vi "high_field_probe_chopper.vi"() -> ()   [LabVIEW 2011]
uses:
  <vilib>/express/express arith-compare/Formula/XNode/ExpressFormulaBlockNode.xnode
  <vilib>/Analysis/NI_AAL_SigProc.lvlib
panel:
  out "Signal":dbl[](graph)
  in  "Set Probe Background":bool
  out "Probe Background":dbl[](graph)
  in  "peak threshold":dbl=0.01 format="%0.2f"
  out "Amplitudes":dbl[](array[numeric])
  in  "Fits?":bool
  out "Waveform Chart 2":dbl(graph)
  out "best fit parameters":dbl[](array[numeric])
  in  "Set Zero Peaks":bool
  out "Peak 2 Amp":dbl
  out "Peak 1 Amp":dbl
  out "Polarization":dbl
  out "Peak Ratio":dbl
  out "XY Graph":cluster{dbl[], dbl[]}[](graph)
  in  "Peak 2 at Zero":dbl=1.0
  in  "Peak 1 at Zero":dbl=1.0
  in  "fit parameters":dbl[](array[numeric])=[0.02, 0.3, 0.12, 0.005, 0.13, 0.012, 0.03, 1.4, 0.12]
  in  "stop":bool
  in  "Center Freq":dbl=1000.0
  in  "Voltage Sweep Range":i32=2
  out "Current Set Voltage":dbl
  in  "threshold":dbl=0.0005
  in  "rate":dbl=20000.0
  in  "number of samples":i32=500
  out "data":dynamicdata(graph)
  out "Waveform Chart":dbl(graph)
  out "amplitude":dbl
  out "frequency":dbl
  # "Height"
  # "Position"
  # "Width"
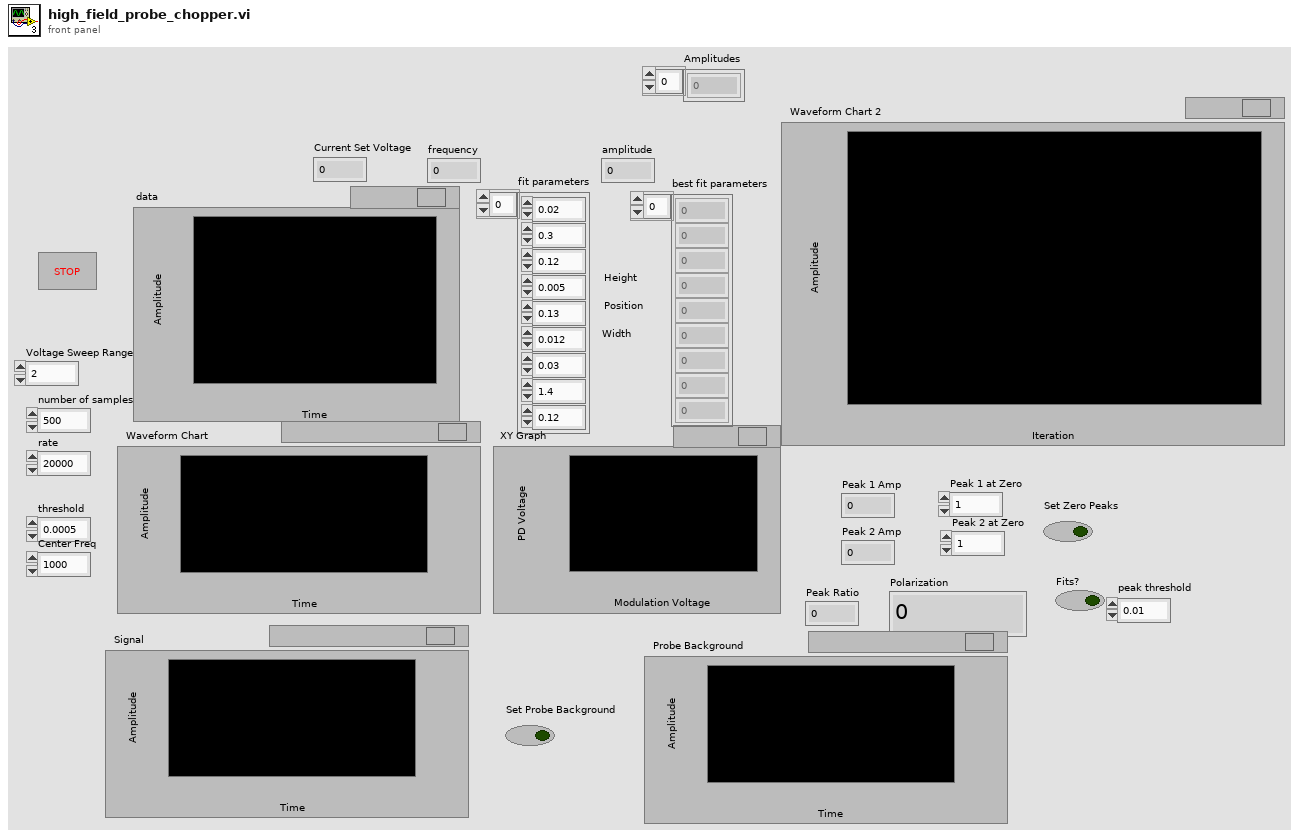
[diagram p1: front panel]
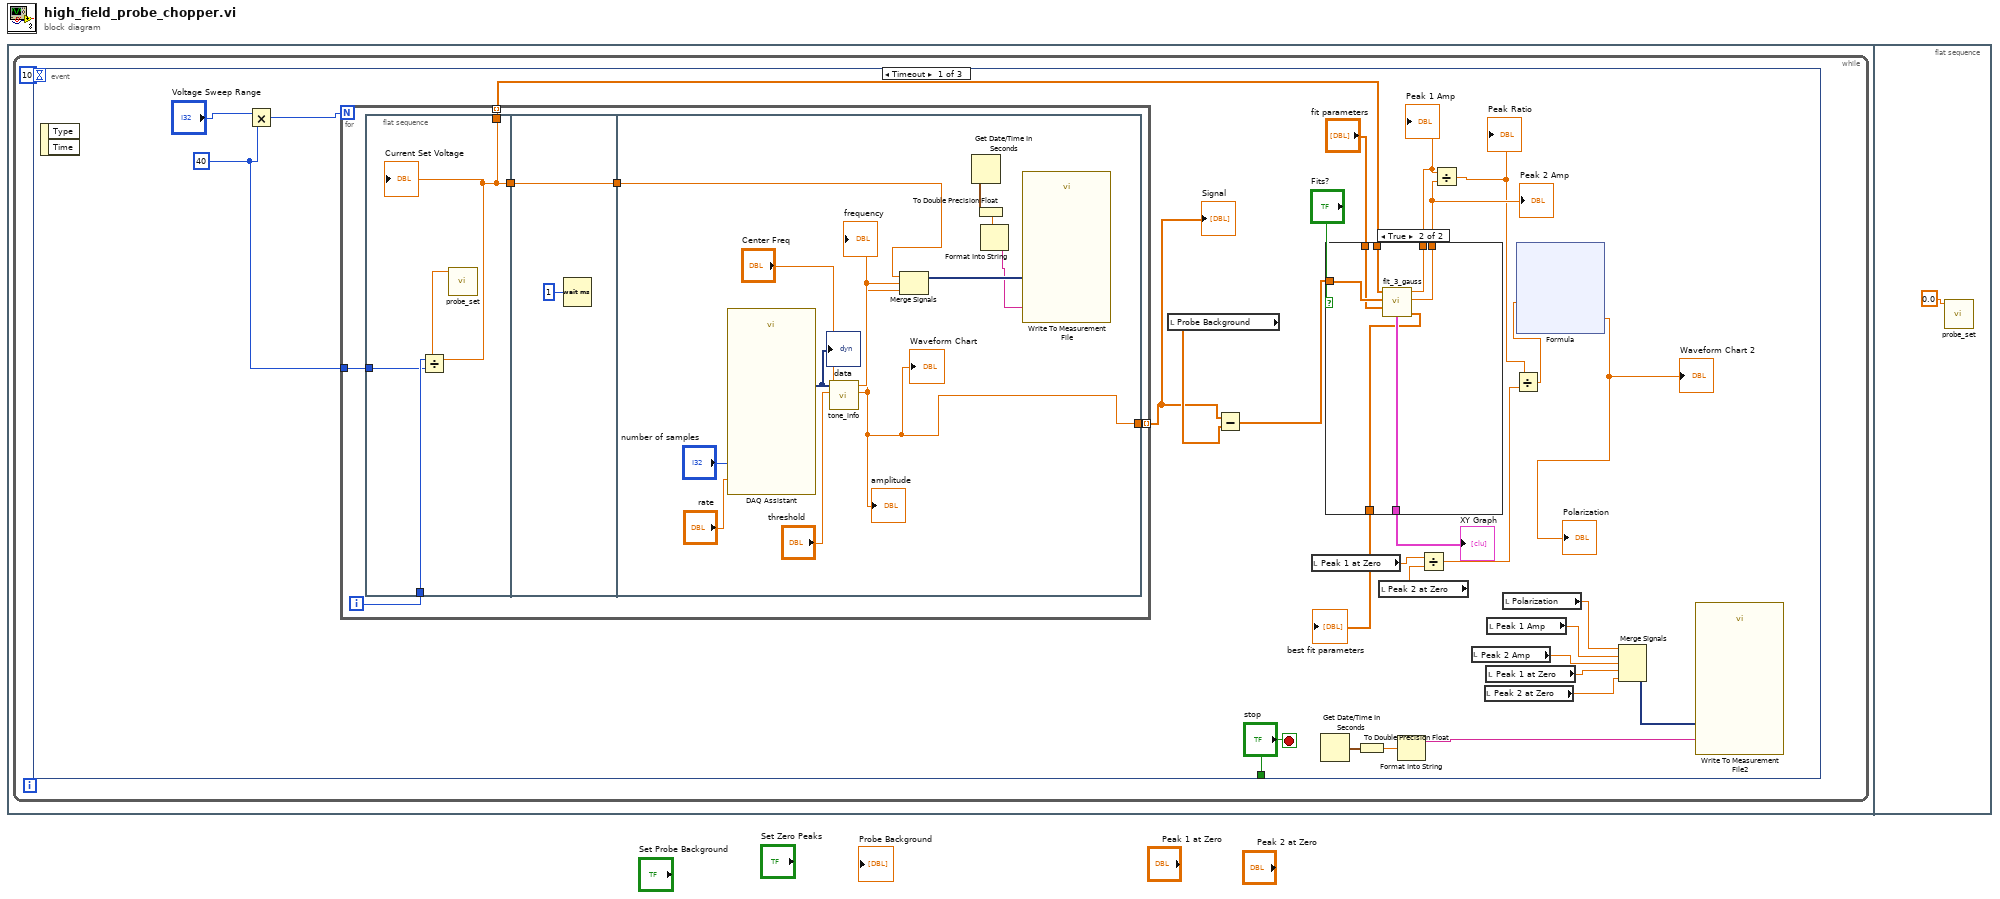
[diagram p0: block diagram]
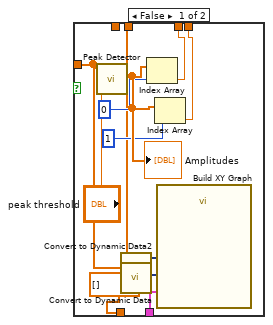
[diagram p2: hidden frame]
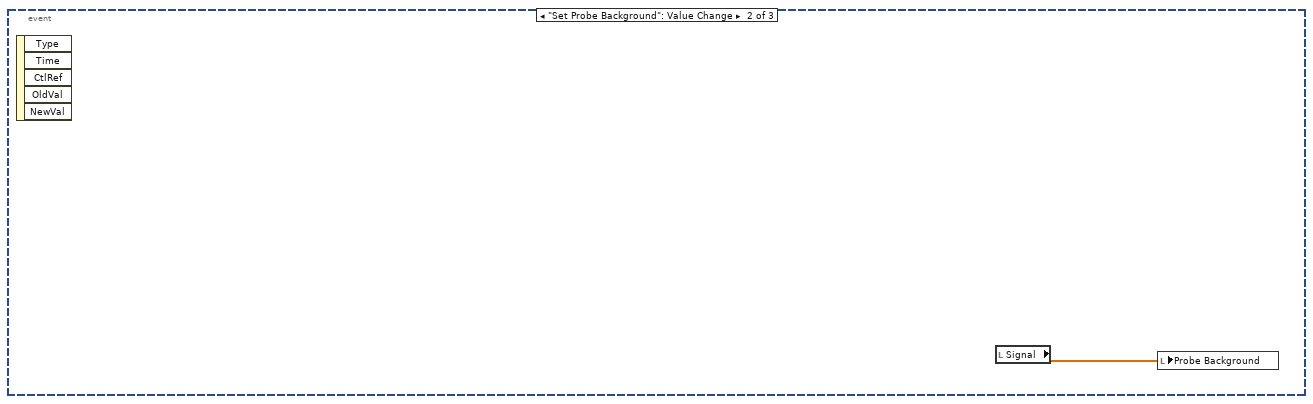
[diagram p3: hidden frame]
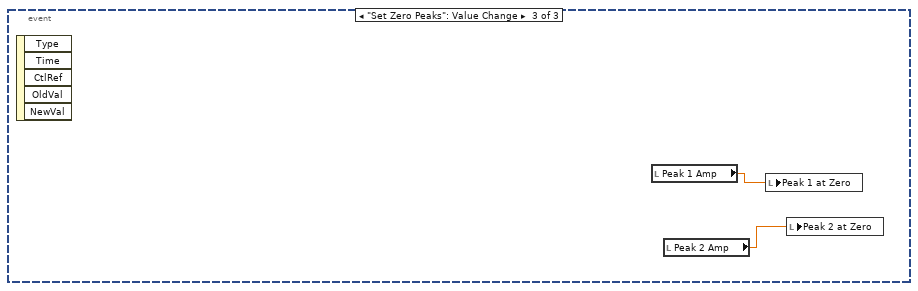
[diagram p4: hidden frame]
diagram:
  n1 = flat-sequence {
    frame #0 {
      n2 = while {
        stop <- w2 stop-if-true
        n3 = event shown="[0] Timeout" {
          selector: _ -> [_ _ _]
          dyn-events: _ -> [_ _ _]
          timeout: 10 -> [_ _ _]
          tunnel: ["stop" _ _] -> w2
          event Timeout {
            w29 = 40 ("y")
            n4 = event-data() -> ()  [unwired: 1 in, 2 out]
            n5 = Multiply(x="Voltage Sweep Range", y=w29) -> (x*y=w30:i32)
            n6 = for {
              N: w30 -> [_]
              tunnel: w29 -> [w63]
              tunnel: [w60] -> w26 mode=indexing
              tunnel: [w59] -> w4 mode=indexing
              i -> [w64]
              n7 = flat-sequence {
                tunnel: w64 -> [w67]
                tunnel: w63 -> [w66]
                tunnel: [w65] -> w61
                tunnel: [w65] -> w60
                tunnel: [w68] -> w62
                tunnel: w61 -> [w68]
                tunnel: w62 -> [w74]
                tunnel: [w70] -> w59
                frame #0 {
                  n8 = Divide(x=w67, y=w66) -> (x/y=w65:dbl)
                  "Current Set Voltage" <- w65
                  n9 = call "probe_set.vi"("Voltage"=w65) -> ()  [unwired: 11 in]
                }
                frame #1 {
                  n10 = Wait (ms)(milliseconds to wait=u32 1) -> ()  [unwired: 1 out]
                }
                frame #2 {
                  n11 = call "DAQ Assistant"("rate"="rate", "number of samples"="number of samples") -> ("data"=w77:dynamicdata)  [unwired: 15 in, 2 out]
                  "data" <- w77
                  n12 = call "tone_info.vi"("Center Freq"="Center Freq", "threshold"="threshold", "time signal in"=w77) -> ("amplitude"=w70:dbl, "frequency"=w81:dbl)  [unwired: 6 in, 1 out]
                  "frequency" <- w81
                  "amplitude" <- w70
                  "Waveform Chart" <- w70
                  n13 = Merge Signals(w74, w81, w70) -> (w76:dynamicdata)
                  n14 = Get Date/Time In Seconds() -> (seconds since 1Jan1904=w73:timestamp)
                  n15 = To Double Precision Float(number=w73) -> (double precision float=w72:dbl)
                  n16 = Format Into String(w72) -> (resulting string=w71:string)  [unwired: 3 in, 1 out]
                  n17 = call "Write To Measurement File"("Signals"=w76, "Comment"=w71) -> ()  [unwired: 15 in, 3 out]
                }
              }
            }
            "Signal" <- w4
            n18 = local read "Probe Background"() -> (w5:dbl[])
            n19 = Subtract(x=w4, y=w5) -> (x-y=w3:dbl[])
            n20 = local read "Peak 1 at Zero"() -> (w18:dbl)
            n21 = Get Date/Time In Seconds() -> (seconds since 1Jan1904=w15:timestamp)
            n22 = case shown="True" "Fits?" {
              tunnel: w3 -> [w37 w50]
              tunnel: "fit parameters" -> [_ w49]
              tunnel: w26 -> [w35 w48]
              tunnel: [w39 w47] -> w25
              tunnel: [w38 w46] -> w24
              tunnel: [w33 w45] -> w23
              tunnel: [dbl[] [] ("best fit parameters") w44] -> w13
              frame False {
                n23 = call <vilib>:"Peak Detector.vi"("threshold"="peak threshold", "X"=w37) -> ("Amplitudes"=w42:dbl[])  [unwired: 5 in, 4 out]
                "Amplitudes" <- w42
                n24 = call "Convert to Dynamic Data2"("Array"=w35) -> ("Dynamic Data Type"=w34:dynamicdata)  [unwired: 3 in]
                n25 = call "Convert to Dynamic Data"("Array"=w37) -> ("Dynamic Data Type"=w36:dynamicdata)  [unwired: 3 in]
                n26 = Index Array(array=w42, index=0) -> (element=w39:dbl)
                n27 = Index Array(array=w42, index=1) -> (element=w38:dbl)
                n28 = call "Build XY Graph"("Y Input"=w36, "X Input"=w34) -> ("XY Graph"=w33:cluster{"Y":dbl[], "Y":dbl[]}[])  [unwired: 3 in, 6 out]
              }
              frame True {
                n29 = call "fit_3_gauss.vi"("initial parameters"=w49, "y Array"=w50, "x Array"=w48) -> ("best fit parameters"=w44:dbl[], "XY Graph"=w45:cluster{dbl[], dbl[]}[], "Peak 3 Amp"=w46:dbl, "Peak 1 Amp"=w47:dbl)  [unwired: 5 in]
              }
            }
            "XY Graph" <- w23
            "Peak 1 Amp" <- w25
            "Peak 2 Amp" <- w24
            "best fit parameters" <- w13
            n30 = To Double Precision Float(number=w15) -> (double precision float=w14:dbl)
            n31 = local read "Peak 2 at Zero"() -> (w17:dbl)
            n32 = Format Into String(w14) -> (resulting string=w22:string)  [unwired: 3 in, 1 out]
            n33 = Divide(x=w18, y=w17) -> (x/y=w20:dbl)
            n34 = Divide(x=w25, y=w24) -> (x/y=w21:dbl)
            "Peak Ratio" <- w21
            n35 = local read "Peak 2 Amp"() -> (w9:dbl)
            n36 = local read "Peak 2 at Zero"() -> (w7:dbl)
            n37 = local read "Peak 1 at Zero"() -> (w8:dbl)
            n38 = local read "Peak 1 Amp"() -> (w10:dbl)
            n39 = local read "Polarization"() -> (w11:dbl)
            n40 = Divide(x=w21, y=w20) -> (x/y=w19:dbl)
            n41 = xnode "Formula"("X"=w19) -> ("Result"=→"Polarization" →"Waveform Chart 2":dbl)  [unwired: 1 in, 1 out]
            n42 = Merge Signals(w11, w10, w9, w8, w7) -> (w16:dynamicdata)
            n43 = call "Write To Measurement File2"("Signals"=w16, "Comment"=w22) -> ()  [unwired: 15 in, 3 out]
          }
          event "Set Probe Background": Value Change {
            n44 = event-data() -> ()  [unwired: 1 in, 5 out]
            n45 = local read "Signal"() -> (w82:dbl[])
            n46 = local write "Probe Background"(w82) -> ()
          }
          event "Set Zero Peaks": Value Change {
            n47 = event-data() -> ()  [unwired: 1 in, 5 out]
            n48 = local read "Peak 1 Amp"() -> (w84:dbl)
            n49 = local read "Peak 2 Amp"() -> (w83:dbl)
            n50 = local write "Peak 1 at Zero"(w84) -> ()
            n51 = local write "Peak 2 at Zero"(w83) -> ()
          }
        }
      }
    }
    frame #1 {
      n52 = call "probe_set.vi"("Voltage"=0.0) -> ()  [unwired: 11 in]
    }
  }
